vi "Agilent U2722 - DC Power Output DC Volts.vi"() -> ()   [LabVIEW 2018]
doc: "This example shows how to configure the instrument's output voltage level, over current protection, and over voltage protection. The actual voltage level and actual current level are returned as well as whether over voltage protection (OVP) or over current protection (OCP) has been tripped."
uses:
  <instrlib>/Agilent U2722/Agilent U2722.lvlib
panel:
  in  "Triggered Level (1.0 V)":dbl=1.0
  in  "Output Level (1.0 V)":dbl=1.0
  in  "Current Limit (1.0 uA)":dbl=1e-06
  in  "Voltage Range (0: 2 Volts)":u16(ring) items=["2 Volts", "20 Volts"]
  in  "Channel (1: Channel 1)":u16(ring)=1 items=["Channel 1"=1, "Channel 2"=2, "Channel 3"=3]
  in  "Stop Output":bool
  out "Actual Current Limit (A)":dbl format="%.2f"
  out "Actual Voltage Level (V)":dbl format="%.2f"
  in  "VISA resource name":refnum<visa-resource-name>
  # "(c) 2009-2015 National Instruments.  ALL RIGHTS RESERVED."
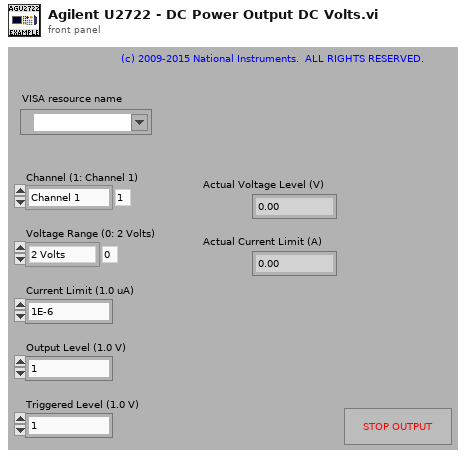
[diagram p1: front panel]
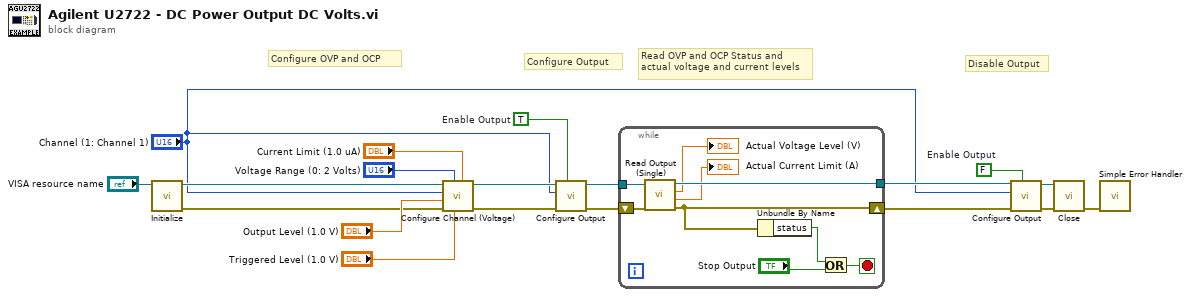
[diagram p0: block diagram]
diagram:
  w9 = TRUE  # Enable Output
  w2 = FALSE  # Enable Output
  # "Disable Output"
  # "Read OVP and OCP Status and\nactual voltage and current levels"
  # "Configure Output"
  # "Configure OVP and OCP"
  n1 = call <instrlib>:"Initialize.vi"("VISA resource name"="VISA resource name") -> ("error out"=w10:errorcluster, "VISA resource name out"=w11:refnum<visa-resource-name>)  [unwired: 9 in]
  n2 = call <instrlib>:"Configure Channel (Voltage).vi"("Voltage Limit (2.0 V)"="Current Limit (1.0 uA)", "Triggered Level (1.0 V)"="Triggered Level (1.0 V)", "Voltage Range (0: 2 Volts)"="Voltage Range (0: 2 Volts)", "error in (no error)"=w10, "Output Level (1.0 V)"="Output Level (1.0 V)", "Channel (1: Channel 1)"="Channel (1: Channel 1)", "VISA resource name"=w11) -> ("error out"=w12:errorcluster, "VISA resource name out"=w13:refnum<visa-resource-name>)  [unwired: 3 in]
  n3 = call <instrlib>:"Configure Output.vi"("Enable Output (T: Enable)"=w9, "error in (no error)"=w12, "Channel (1: Channel 1)"="Channel (1: Channel 1)", "VISA resource name"=w13) -> ("error out"=w7:errorcluster, "VISA resource name out"=w8:refnum<visa-resource-name>)  [unwired: 6 in]
  n4 = while {
    tunnel: w8 -> [w26]
    shift-right: [w21] -> w5
    shift-left: w7 -> [w25]
    tunnel: [w24] -> w6
    stop <- w28 stop-if-true
    n5 = call <instrlib>:"Read Output (Single).vi"("error in (no error)"=w25, "VISA resource name"=w26) -> ("error out"=w21:errorcluster, "Actual Current Level (A)"=→"Actual Current Limit (A)":dbl, "Actual Voltage Level (V)"=→"Actual Voltage Level (V)":dbl, "VISA resource name out"=w24:refnum<visa-resource-name>)  [unwired: 6 in]
    n6 = Unbundle By Name(w21) -> ("status"=w20:bool)
    n7 = Or(x=w20, y="Stop Output") -> (x .or. y?=w28:bool)
  }
  n8 = call <instrlib>:"Configure Output.vi"("Enable Output (T: Enable)"=w2, "error in (no error)"=w5, "Channel (1: Channel 1)"="Channel (1: Channel 1)", "VISA resource name"=w6) -> ("error out"=w3:errorcluster, "VISA resource name out"=w4:refnum<visa-resource-name>)  [unwired: 6 in]
  n9 = call <instrlib>:"Close.vi"("error in (no error)"=w3, "VISA resource name"=w4) -> ("error out"=w19:errorcluster)  [unwired: 9 in]
  n10 = call <vilib>:"Simple Error Handler.vi"("error in (no error)"=w19) -> ()  [unwired: 4 in, 5 out]
